vi "AMX-CCD5 自动处理图像.vi"(5 "All Files in Dir 2":path[](array[path]), 7 "数值 2":i32, 9 "A/B段位置切换":bool, 11 "error in (no error)":errorcluster caption="错误输入（无错误）") -> (0 "Image In":T1(plugin-control), 4 "Image Out":T1(plugin-control), 6 "颗粒物有无判断":bool, 8 "颗粒物大小显示":dbl[](array[numeric]), 10 "颗粒物位置坐标":cluster{"X":dbl, "Y":dbl}[](array[cluster]) {"Y" format="%.2f"; "X" format="%.2f"}, 14 "结果":bool, 15 "error out":errorcluster caption="错误输出")   [LabVIEW 2017]
uses:
  Global System.vi
panel:
  out "处理时间":dbl
  out "结果数组":bool[](array[boolean])
  out "单个图片路径":path
  in  "颗粒物个数阈值":i32
  out "数值":i32
  out "处理完成信号":bool
  out "子字符串":string
  out "处理完成文件":string[](array[string])
  out "All Files in Dir":path[](array[path]) caption="目录中的所有文件"
  out "未处理文件":string[](array[string])
  out "x = y?":bool[](array[boolean])
  out "数值 3":i32
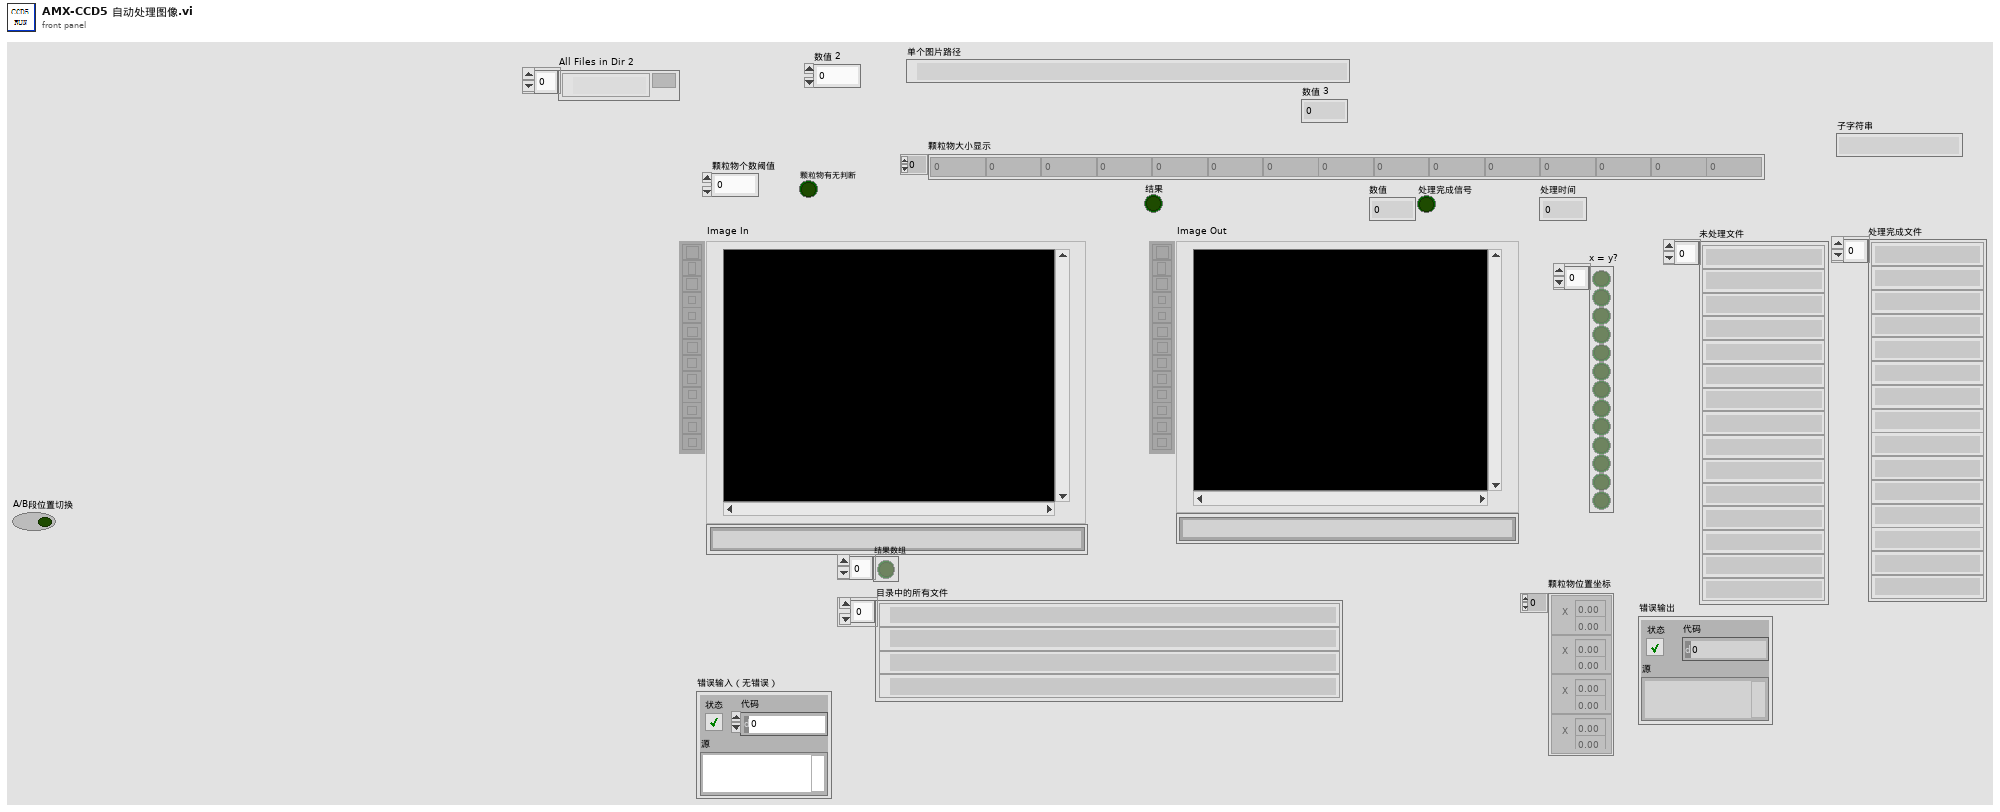
[diagram p1: front panel]
types:
  T1 = typedef "IMAQ Image.ctl" = refnum<image>
  T2 = typedef "IMAQ Rectangle" = cluster{"Left":i32, "Top":i32, "Right":i32, "Bottom":i32, "Rotation":dbl}
  T3 = cluster{"Rectangle":T2, "Threshold Limits (Threshold 1)":cluster{"Lower value":sgl, "Upper value":sgl}, "Keep/Remove Particles ":bool, "Connectivity 4/8 (8) ":bool, "Selection Values (Particle Filter 1)":cluster{"Measurement Parameter":i32, "Range Lower Value":dbl, "Range Upper Value":dbl, "Range":bool, "Measurement Type":bool}[], "Corner Options (Feature Detection 1)":cluster{"Detector type":enum32{"Harris Corner", "Shi-Tomasi Corner"}, "Kernel size":i32, "Min Corner Point Strength":dbl}, "Pyramid level (Feature Detection 1)":u32, "Method ":i32, "Look For":u32, "Method 2":i32, "ROI Descriptor (Clamp (Rake) 1)":cluster{"Global Rectangle":i32[], "Contours":cluster{"ID":enum32{"External", "Internal"}, "Type":u32, "Coordinates":i32[]}[]}}
  T4 = typedef "IMAQ Curve Parameters.ctl" = cluster{"Extraction Mode":u32, "Edge Threshold":i32, "Edge Filter Size":u32, "Min Length":i32, "Row Search Step Size":i32, "Col Search Step Size":i32, "Max Endpoint Gap":i32, "Closed":bool, "Subpixel":bool}
  T5 = cluster{"Curve Extraction Settings ":T4, "Color Mode (Histogram 1)":u16, "Range (Threshold 1)":cluster{"Lower value":sgl, "Upper value":sgl}, "Clamp Settings (Max Clamp 1)":cluster{"Angle Range (+/-)":dbl, "Edge Polarity":cluster{"Start":u32, "End":u32}}, "Settings (Clamp (Rake) 1)":cluster{"Contrast":i32, "Filter width":i32, "Steepness":i32, "Subsampling Ratio":u32, "Show Search Area":bool, "Show Search Lines":bool, "Show Edges Found":bool, "Show Result":bool}, "直径设定":cluster{"Lower value":sgl, "Upper value":sgl}}
  T6 = typedef "Image Type" = u32
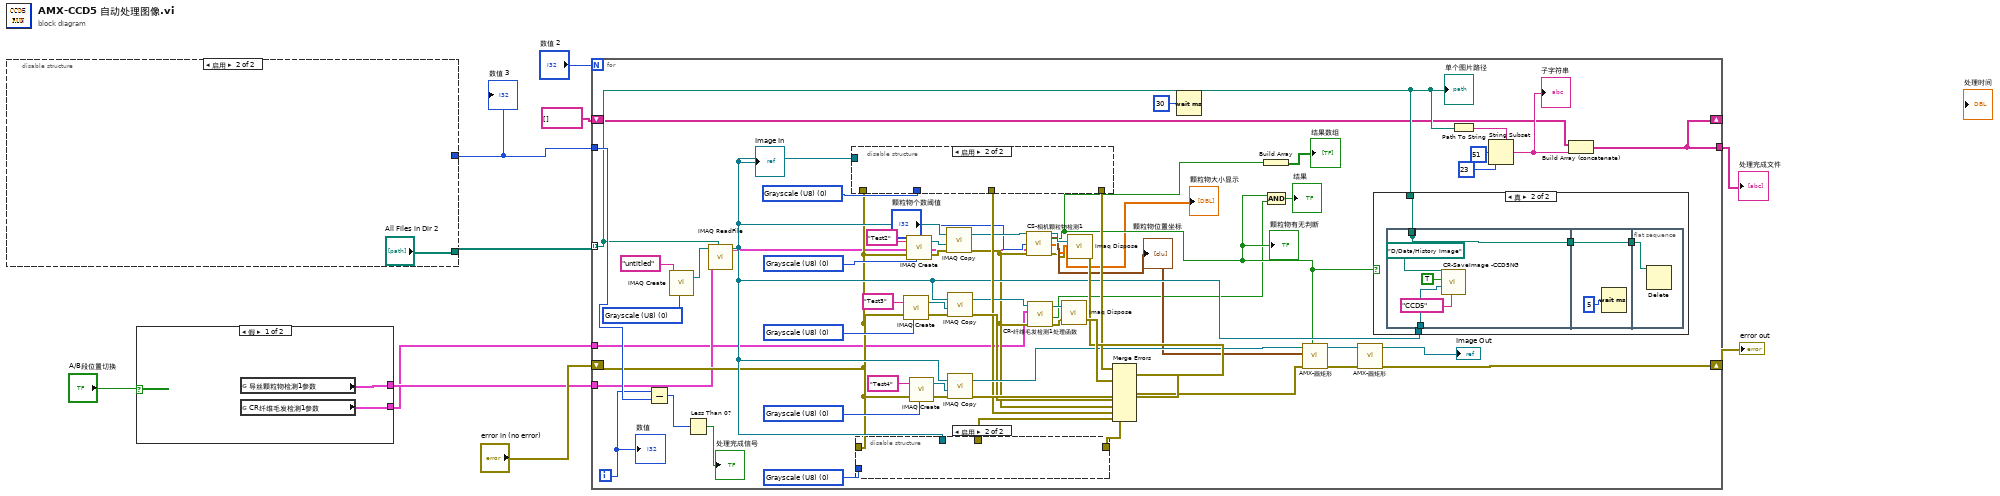
[diagram p0: block diagram]
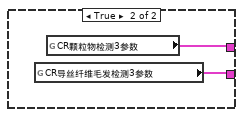
[diagram p2: hidden frame]
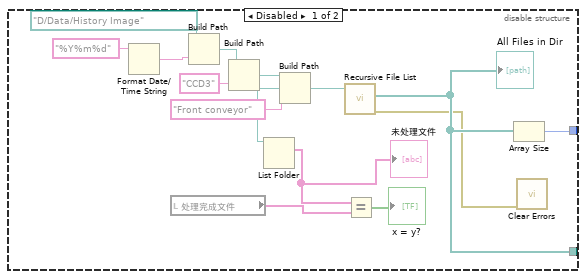
[diagram p3: hidden frame]
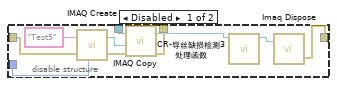
[diagram p4: hidden frame]
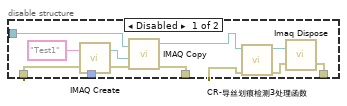
[diagram p5: hidden frame]
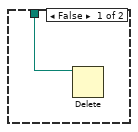
[diagram p6: hidden frame]
diagram:
  n1 = disable-structure shown="启用" {
    disable-tunnel: [w17 _] -> w9
    disable-tunnel: [w16 "All Files in Dir 2"] -> w8
    frame Disabled {
      n2 = Format Date/Time String(time format string (%c)="%Y%m%d" ("时间格式字符串(%c)")) -> (date/time string=w18:string)  [unwired: 2 in]
      n3 = local read "处理完成文件"() -> (w13:string[])
      n4 = Build Path(base path=path "D:/Data/History Image" ("基路径"), name or relative path=w18) -> (appended path=w21:path)
      n5 = Build Path(base path=w21, name or relative path="CCD3" ("名称或相对路径")) -> (appended path=w19:path)
      n6 = Build Path(base path=w19, name or relative path="Front conveyor" ("名称或相对路径")) -> (appended path=w15:path)
      n7 = List Folder(path=w15) -> (filenames=w14:string[])  [unwired: 3 in, 3 out]
      "未处理文件" <- w14
      n8 = call <vilib>:"Recursive File List.vi"("Folder Path"=w15) -> ("error out"=w11:errorcluster, "All Files in Dir"=w16:path[])  [unwired: 6 in, 3 out]
      "All Files in Dir" <- w16
      n9 = Equal?(x=w14, y=w13) -> (x = y?=→"x = y?":bool[])
      n10 = Array Size(array=w16) -> (size(s)=w17:i32)
      n11 = call <vilib>:"Clear Errors.vi"("error in (no error)"=w11) -> ()  [unwired: 5 in, 2 out]
    }
    frame Enabled {
    }
  }
  "数值 3" <- w9
  n12 = case shown="假" "A/B段位置切换" {
    tunnel: [w27 w29] -> w2
    tunnel: [w26 w28] -> w1
    frame False {
      n13 = global read "Global System.vi" "导丝颗粒物检测1参数"() -> (w27:T3)
      n14 = global read "Global System.vi" "CR纤维毛发检测1参数"() -> (w26:T5)
    }
    frame True {
      n15 = global read "Global System.vi" "CR导丝纤维毛发检测3参数"() -> (w28:T5)
      n16 = global read "Global System.vi" "CR颗粒物检测3参数"() -> (w29:T3)
    }
  }
  n17 = for {
    N: "数值 2" -> [_]
    tunnel: w8 -> [w56] mode=indexing
    shift-right: [w90] -> w7
    shift-left: "error in (no error)" -> [w43]
    tunnel: w9 -> [w58]
    shift-right: [w50] -> _
    shift-left: string[] [] ("添加的数组") -> [w51]
    tunnel: [w50] -> w5
    tunnel: w2 -> [w31]
    tunnel: w1 -> [w30]
    i -> [w57]
    w62 = T6 0 items=["Grayscale (U8)", "Grayscale (I16)", "Grayscale (SGL)", "Complex (CSG)", "RGB (U32)", "HSL (U32)", "RGB (U64)", "Grayscale (U16)"] ("Image Type")
    w66 = T6 0 items=["Grayscale (U8)", "Grayscale (I16)", "Grayscale (SGL)", "Complex (CSG)", "RGB (U32)", "HSL (U32)", "RGB (U64)", "Grayscale (U16)"] ("Image Type")
    w67 = T6 0 items=["Grayscale (U8)", "Grayscale (I16)", "Grayscale (SGL)", "Complex (CSG)", "RGB (U32)", "HSL (U32)", "RGB (U64)", "Grayscale (U16)"] ("Image Type")
    w69 = T6 0 items=["Grayscale (U8)", "Grayscale (I16)", "Grayscale (SGL)", "Complex (CSG)", "RGB (U32)", "HSL (U32)", "RGB (U64)", "Grayscale (U16)"] ("Image Type")
    w75 = T6 0 items=["Grayscale (U8)", "Grayscale (I16)", "Grayscale (SGL)", "Complex (CSG)", "RGB (U32)", "HSL (U32)", "RGB (U64)", "Grayscale (U16)"] ("Image Type")
    w76 = T6 0 items=["Grayscale (U8)", "Grayscale (I16)", "Grayscale (SGL)", "Complex (CSG)", "RGB (U32)", "HSL (U32)", "RGB (U64)", "Grayscale (U16)"] ("Image Type")
    n18 = Subtract(x=w57, y=w58) -> (x-y=w60:i32)
    n19 = call "IMAQ Create"("Image Name"="untitled", "Image Type"=w76) -> ("New Image"=w78:T1)  [unwired: 3 in, 1 out]
    n20 = Less Than 0?(x=w60) -> (x < 0?=→"处理完成信号":bool)
    n21 = call "IMAQ ReadFile"("File Path"=w56, "Image"=w78) -> ("Image Out"=w46:T1)  [unwired: 5 in, 4 out]
    "Image In" <- w46
    n22 = disable-structure shown="启用" {
      disable-tunnel: [w111 _] -> w82
      disable-tunnel: w62 -> [w110 _]
      disable-tunnel: [w106 _] -> w48
      disable-tunnel: w46 -> [w105 _]
      disable-tunnel: w43 -> [w102 _]
      frame Disabled {
        n23 = call "IMAQ Create"("Image Name"="Test1", "Image Type"=w110, "error in (no error)"=w102) -> ("New Image"=w108:T1, "error out"=w109:errorcluster)  [unwired: 2 in]
        n24 = call "IMAQ Copy"("error in (no error)"=w109, "Image Dst"=w108, "Image Src"=w105) -> ("error out"=w106:errorcluster, "Image Dst Out"=w104:T1)  [unwired: 3 in]
        n25 = call "CR-导丝划痕检测3处理函数.vi"("error in (no error)"=w102, "Image in"=w104) -> ("error out"=w101:errorcluster, "Image out"=w103:T1)  [unwired: 6 in, 2 out]
        n26 = call "Imaq Dispose"("Image"=w103, "error in (no error)"=w101) -> ("error out"=w111:errorcluster)  [unwired: 4 in]
      }
      frame Enabled {
      }
    }
    n27 = disable-structure shown="启用" {
      disable-tunnel: [w100 _] -> w85
      disable-tunnel: w67 -> [w98 _]
      disable-tunnel: [w95 _] -> w47
      disable-tunnel: w46 -> [w94 _]
      disable-tunnel: w43 -> [w91 _]
      frame Disabled {
        n28 = call "IMAQ Create"("Image Name"="Test5", "Image Type"=w98, "error in (no error)"=w91) -> ("New Image"=w97:T1, "error out"=w96:errorcluster)  [unwired: 2 in]
        n29 = call "IMAQ Copy"("error in (no error)"=w96, "Image Dst"=w97, "Image Src"=w94) -> ("error out"=w95:errorcluster, "Image Dst Out"=w93:T1)  [unwired: 3 in]
        n30 = call "CR-导丝缺损检测3处理函数.vi"("Image in"=w93) -> ("Image out"=w92:T1)  [unwired: 7 in, 3 out]
        n31 = call "Imaq Dispose"("Image"=w92) -> ("error out"=w100:errorcluster)  [unwired: 5 in]
      }
      frame Enabled {
      }
    }
    n32 = call "IMAQ Create"("Image Name"="Test3", "Image Type"=w66, "error in (no error)"=w43) -> ("New Image"=w64:T1, "error out"=w63:errorcluster)  [unwired: 2 in]
    n33 = call "IMAQ Create"("Image Name"="Test2", "Image Type"=w75, "error in (no error)"=w43) -> ("New Image"=w73:T1, "error out"=w72:errorcluster)  [unwired: 2 in]
    n34 = call "IMAQ Create"("Image Name"="Test4", "Image Type"=w69, "error in (no error)"=w43) -> ("New Image"=w70:T1, "error out"=w71:errorcluster)  [unwired: 2 in]
    n35 = call "IMAQ Copy"("error in (no error)"=w72, "Image Dst"=w73, "Image Src"=w46) -> ("error out"=w33:errorcluster, "Image Dst Out"=w42:T1)  [unwired: 3 in]
    n36 = call "IMAQ Copy"("error in (no error)"=w63, "Image Dst"=w64, "Image Src"=w46) -> ("error out"=w49:errorcluster, "Image Dst Out"=w45:T1)  [unwired: 3 in]
    n37 = call "IMAQ Copy"("error in (no error)"=w71, "Image Dst"=w70, "Image Src"=w46) -> ("error out"=w87:errorcluster, "Image Dst Out"=w80:T1)  [unwired: 3 in]
    n38 = call "CS-相机颗粒物检测1.vi"("Image in"=w42, "颗粒物个数阈值"="颗粒物个数阈值", "导丝颗粒物检测1参数"=w31, "error in (no error)"=w33) -> ("颗粒物位置坐标"=w38:cluster{"X":dbl, "Y":dbl}[], "Image out"=w40:T1, "颗粒物有无显示"=w39:bool, "颗粒物大小显示"=→"颗粒物大小显示":dbl[], "error out"=w32:errorcluster)  [unwired: 5 in, 2 out]
    "颗粒物有无判断" <- w39
    "颗粒物位置坐标" <- w38
    n39 = call "CR-纤维毛发检测1处理函数.vi"("error in (no error)"=w33, "UI电源线正面漏线参数"=w30, "Image in"=w45) -> ("error out"=w34:errorcluster, "纤维毛发"=w36:bool, "Image out"=w44:T1)  [unwired: 4 in, 2 out]
    n40 = call "Imaq Dispose"("Image"=w44, "error in (no error)"=w34) -> ("error out"=w84:errorcluster)  [unwired: 4 in]
    n41 = call "Imaq Dispose"("Image"=w40, "error in (no error)"=w32) -> ("error out"=w83:errorcluster)  [unwired: 4 in]
    n42 = Merge Errors(w82, w83, w84, w87, w85, w49, w33, w48, w47) -> (w81:errorcluster)
    n43 = Wait (ms)(milliseconds to wait=u32 30 ("等待时间（毫秒）")) -> ()  [unwired: 1 out]
    n44 = Build Array(w39) -> (→"结果数组":bool[])
    n45 = Compound Arithmetic op=AND ("复合运算")(w39, w36) -> (→"结果":bool)
    n46 = call "AMX-画矩形.vi"("布尔"=w39, "error in (no error)"=w81, "颗粒物位置坐标"=w38, "Image In"=w80) -> ("error out"=w88:errorcluster, "Image Out"=w89:T1)  [unwired: 6 in]
    n47 = call "AMX-画矩形.vi"("error in (no error)"=w88, "Image In"=w89) -> ("error out"=w90:errorcluster, "Image Out"=→"Image Out":T1)  [unwired: 8 in]
    n48 = case shown="真" w39 {
      tunnel: w56 -> [w112 w115]
      tunnel: w46 -> [_ w116]
      frame False {
        n49 = Delete(path (use dialog)=w112) -> ()  [unwired: 4 in, 3 out]
      }
      frame True {
        n50 = flat-sequence {
          tunnel: w116 -> [w121]
          tunnel: [w117] -> _
          tunnel: w115 -> [w117]
          tunnel: [w117] -> w114
          tunnel: w114 -> [w122]
          tunnel: [w122] -> w113
          tunnel: w113 -> [w124]
          frame #0 {
            n51 = call "CR-SaveImage -CCD5NG.vi"("CCD Name"="CCD5", "Image in"=w121, "布尔"=TRUE, "基路径"=path "D:/Data/History Image") -> ()  [unwired: 7 in, 1 out]
          }
          frame #1 {
            n52 = Wait (ms)(milliseconds to wait=u32 5 ("等待时间（毫秒）")) -> ()  [unwired: 1 out]
          }
          frame #2 {
            n53 = Delete(path (use dialog)=w124) -> ()  [unwired: 4 in, 3 out]
          }
        }
      }
    }
    n54 = Path To String(path=w56) -> (string=w55:string)
    n55 = String Subset(string=w55, offset (0)=51 ("偏移量(0)"), length (rest)=23 ("长度（剩余）")) -> (substring=w52:string)
    "子字符串" <- w52
    n56 = Build Array (concatenate)(w51, w52) -> (w50:string[])
    "单个图片路径" <- w56
    "数值" <- w57
  }
  "error out" <- w7
  "处理完成文件" <- w5
